vi "Read ADC.vi"(8 "Valor pin":string(combo), 9 "PIN":i32, 10 "CH":i32, 11 "Serial Devide Brand":T1) -> (2 "Expected Response":string, 3 "Command to Send":string)   [LabVIEW 2020]
uses:
  Combo Box Devices.ctl
  Combo Box Comandos.ctl
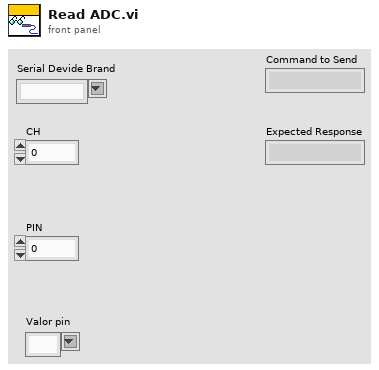
[diagram p1: front panel]
types:
  T1 = typedef "Combo Box Devices.ctl" = string
  T2 = typedef "Combo Box Comandos.ctl" = string
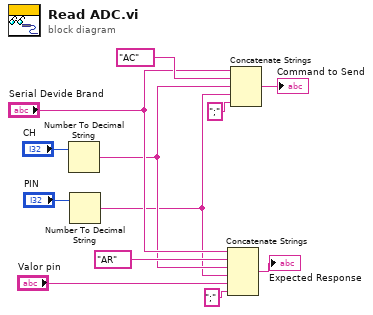
[diagram p0: block diagram]
diagram:
  n1 = Number To Decimal String(number="CH") -> (decimal integer string=w6:string)  [unwired: 1 in]
  n2 = Number To Decimal String(number="PIN") -> (decimal integer string=w3:string)  [unwired: 1 in]
  n3 = Concatenate Strings("Serial Devide Brand", T2 "AR" ("Respuesta"), w6, w3, "Valor pin", ";" ("string")) -> (→"Expected Response":string)
  n4 = Concatenate Strings("Serial Devide Brand", T2 "AC" ("Command"), w6, w3, ";" ("string")) -> (→"Command to Send":string)
